vi "XW_Map_Wrapper_Test_Trimesh_PN.vi"() -> ()   [LabVIEW 2011]
uses:
  Qtree vis/Trimmed down TreeNode2D.ctl
panel:
  out "All nodes processed and processed without error":bool=TRUE
  in  "Domain padding factor":dbl=1.01
  in  "Apply calibration corrections":bool
  in  "n2 from Vel. Calib":dbl=0.41
  in  "B2 from Vel. Calib":dbl=1.4
  in  "A2 from Vel. Calib":dbl=2.25
  in  "n1 from Vel. Calib":dbl=0.42
  in  "B1 from Vel. Calib":dbl=1.36
  in  "A1 from Vel. Calib":dbl=2.21
  out "V (m/s)":dbl=2.628922027659496
  out "U (m/s)":dbl=8.536690147950912
  out "Voltages are inside calibrated region":bool=TRUE
  in  "(E1 / G1) + O1 (Volts)":dbl=2.4
  in  "(E2 / G2) + O2 (Volts)":dbl=2.2
  in  "XW_Calib_Map file path (dialog if empty)":path=path "C:/Documents and Settings/Paul Nathan/Desktop/XW Calib Map/XW Calib Map TRIMESH vi/XW_Map_Wire001OH65_080210.txt"
  # "Paul Nathan 17/02/10"
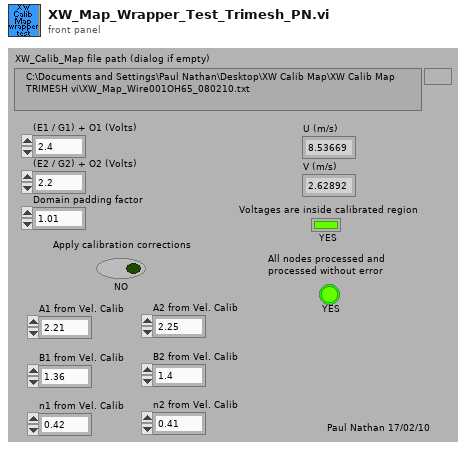
[diagram p1: front panel]
types:
  T1 = typedef "Trimmed down TreeNode2D.ctl" = cluster{"Xmax":dbl, "Xmin":dbl, "Ymax":dbl, "Ymin":dbl, "Xc":dbl, "Yc":dbl, "ObjIndexList":i32[], "NodeQ1Index":i32, "NodeQ2Index":i32, "NodeQ3Index":i32, "NodeQ4Index":i32}
  T2 = typedef "Triangle2D.ctl" = cluster{"V10":dbl[], "V20":dbl[], "1/det":dbl, "V0":cluster{"PosVector":dbl[], "ValueVector":dbl[]}, "V1":cluster{"PosVector":dbl[], "ValueVector":dbl[]}, "V2":cluster{"PosVector":dbl[], "ValueVector":dbl[]}, "V21":dbl[]}
  T3 = typedef "TreeNode2D.ctl" = cluster{"Xmax":dbl, "Xmin":dbl, "Ymax":dbl, "Ymin":dbl, "Xc":dbl, "Yc":dbl, "Px":dbl, "Py":dbl, "q":dbl, "Level":i32, "ObjIndexList":i32[], "ParentIndex":i32, "NodeQ1Index":i32, "NodeQ2Index":i32, "NodeQ3Index":i32, "NodeQ4Index":i32, "EdgeVectorsQ1":dbl[][], "EdgeVectorsQ2":dbl[][], "EdgeVectorsQ3":dbl[][], "EdgeVectorsQ4":dbl[][], "PointOnEdgeVectorsQ1":dbl[][], "PointOnEdgeVectorsQ2":dbl[][], "PointOnEdgeVectorsQ3":dbl[][], "PointOnEdgeVectorsQ4":dbl[][]}
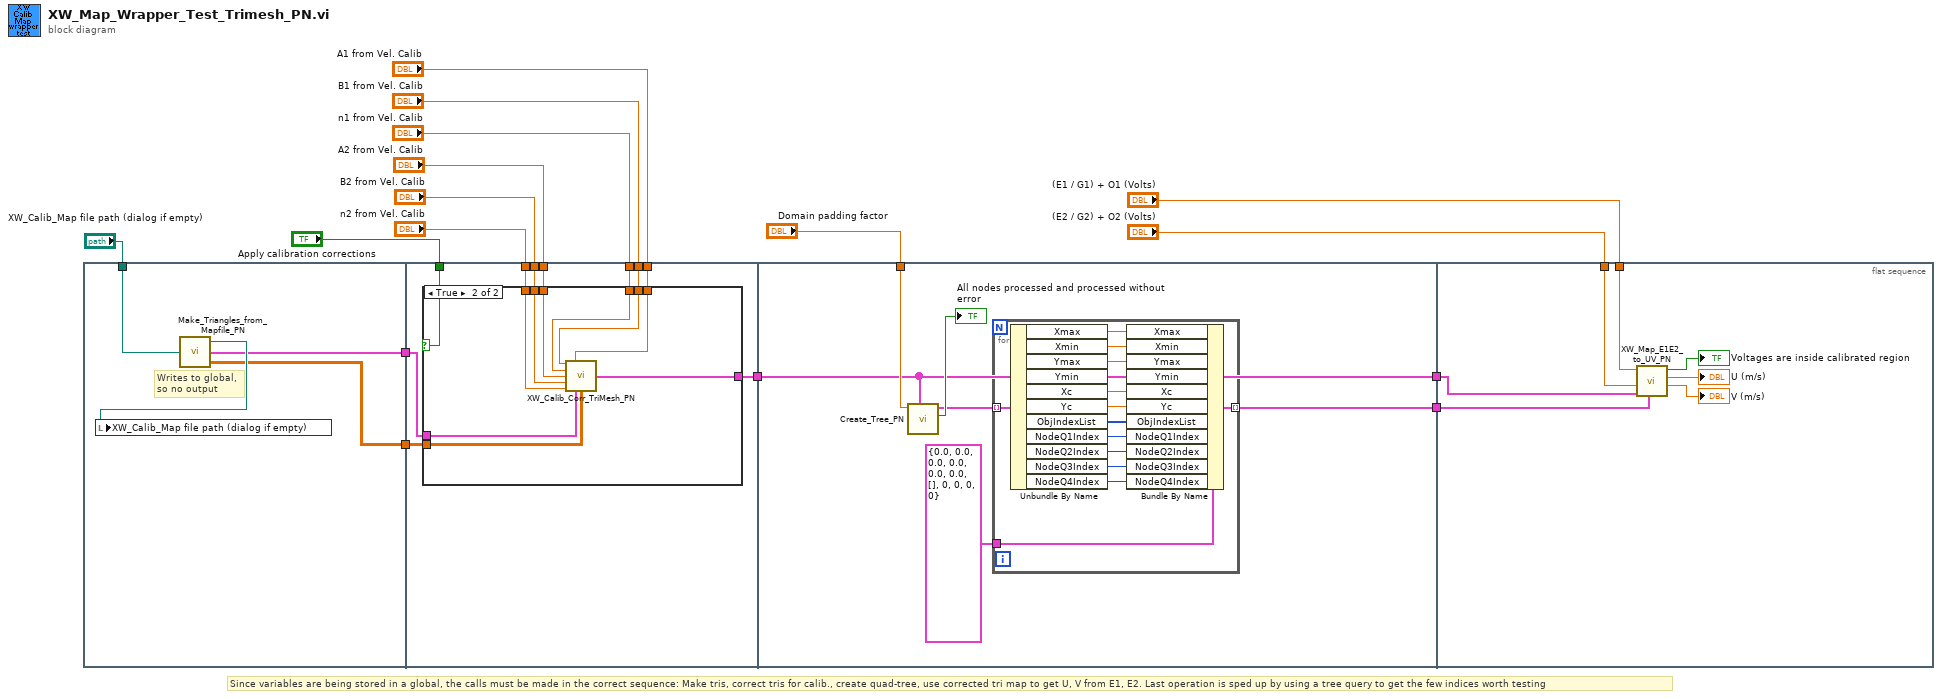
[diagram p0: block diagram]
diagram:
  # "Since variables are being stored in a global, the calls must be made in the correct sequence: Make tris, correct tris for calib., create quad-tree, use corrected tri map to get U, V from E1, E2. Last operation is sped up by using a tree query to get the few indices worth testing"
  n1 = flat-sequence {
    tunnel: "XW_Calib_Map file path (dialog if empty)" -> [w20]
    tunnel: [w18] -> w3
    tunnel: [w17] -> w2
    tunnel: "Apply calibration corrections" -> [w30]
    tunnel: "n2 from Vel. Calib" -> [w29]
    tunnel: "B2 from Vel. Calib" -> [w28]
    tunnel: "A2 from Vel. Calib" -> [w27]
    tunnel: "n1 from Vel. Calib" -> [w26]
    tunnel: "B1 from Vel. Calib" -> [w25]
    tunnel: "A1 from Vel. Calib" -> [w24]
    tunnel: [w23] -> w4
    tunnel: w3 -> [w22]
    tunnel: w2 -> [w21]
    tunnel: "Domain padding factor" -> [w46]
    tunnel: [w42] -> w5
    tunnel: w4 -> [w41]
    tunnel: [w41] -> w1
    tunnel: "(E2 / G2) + O2 (Volts)" -> [w64]
    tunnel: "(E1 / G1) + O1 (Volts)" -> [w63]
    tunnel: w5 -> [w62]
    tunnel: w1 -> [w61]
    frame #0 {
      # "Writes to global,\nso no output"
      n2 = call "Make_Triangles_from_Mapfile_PN.vi"("XW_Calib_Map file path (dialog if empty)"=w20) -> ("XW_Calib_Map file path"=w19:path, "Triangles"=w18:T2[], "Zero angle dataset from map (used for calib. correction)"=w17:dbl[][])
      n3 = local write "XW_Calib_Map file path (dialog if empty)"(w19) -> ()
    }
    frame #1 {
      n4 = case shown="True" w30 {
        tunnel: w29 -> [_ w35]
        tunnel: w28 -> [_ w36]
        tunnel: w27 -> [_ w37]
        tunnel: w26 -> [_ w40]
        tunnel: w25 -> [_ w39]
        tunnel: w24 -> [_ w38]
        tunnel: [w31 w34] -> w23
        tunnel: w22 -> [w31 w33]
        tunnel: w21 -> [_ w32]
        frame False {
          # "if not correcting, then set\ncorrected tris equal to\noriginal tris for use"
        }
        frame True {
          n5 = call "XW_Calib_Corr_TriMesh_PN.vi"("B1 from Vel. Calib"=w39, "A1 from Vel. Calib"=w38, "n1 from Vel. Calib"=w40, "A2 from Vel. Calib"=w37, "B2 from Vel. Calib"=w36, "n2 from Vel. Calib"=w35, "Original triangles"=w33, "Zero angle dataset from map (used for calib. correction)"=w32) -> ("Corrected triangles"=w34:T2[])  [unwired: 7 out]
        }
      }
    }
    frame #2 {
      n6 = call "Create_Tree_PN.vi"("Triangles"=w41, "Pad"=w46) -> ("All nodes processed and processed without error"=→"All nodes processed and processed without error":bool, "TreeNodes out"=w43:T3[])  [unwired: 3 in, 2 out]
      n7 = for {
        tunnel: w43 -> [w60] mode=indexing
        tunnel: [w58] -> w42 mode=indexing
        tunnel: T1 {"Xmax"=0.0, "Xmin"=0.0, "Ymax"=0.0, "Ymin"=0.0, "Xc"=0.0, "Yc"=0.0, "ObjIndexList"=[], "NodeQ1Index"=0, "NodeQ2Index"=0, "NodeQ3Index"=0, "NodeQ4Index"=0} ("Trimmed down TreeNode") -> [w59]
        n8 = Unbundle By Name(w60) -> ("Xmax"=w57:dbl, "Xmin"=w56:dbl, "Ymax"=w55:dbl, "Ymin"=w54:dbl, "Xc"=w53:dbl, "Yc"=w52:dbl, "ObjIndexList"=w51:i32[], "NodeQ1Index"=w50:i32, "NodeQ2Index"=w49:i32, "NodeQ3Index"=w48:i32, "NodeQ4Index"=w47:i32)
        n9 = Bundle By Name(cluster=w59, "Xmax"=w57, "Xmin"=w56, "Ymax"=w55, "Ymin"=w54, "Xc"=w53, "Yc"=w52, "ObjIndexList"=w51, "NodeQ1Index"=w50, "NodeQ2Index"=w49, "NodeQ3Index"=w48, "NodeQ4Index"=w47) -> (w58:T1)
      }
    }
    frame #3 {
      n10 = call "XW_Map_E1E2_to_UV_PN.vi"("Trimmed down TreeNode array"=w62, "Triangulated XW Calib Map Mesh"=w61, "(E2 / G2) + O2 (Volts)"=w64, "(E1 / G1) + O1 (Volts)"=w63) -> ("V (m/s)"=→"V (m/s)":dbl, "U (m/s)"=→"U (m/s)":dbl, "Voltages are inside calibrated region"=→"Voltages are inside calibrated region":bool)  [unwired: 5 out]
    }
  }
